vi "SRQ Mode.vi"(8 "error in (no error)":errorcluster, 9 "srq (0:off)":u16(ring) items=["off", "all output faults", "error conditions", "both fault and error conditions"], 11 "VISA resource name":refnum<visa-resource-name>) -> (0 "error out":errorcluster, 3 "VISA resource name out":refnum<visa-resource-name>)   [LabVIEW 2020, in "Agilent 6XXX Series.lvlib"]
doc: "This function enables or disables the SRQ feature for the HP662XA series only."
uses:
  <instrlib>/Agilent 6XXX Series/Agilent 6XXX Series.lvlib
panel:
  # "HP662XA series only"
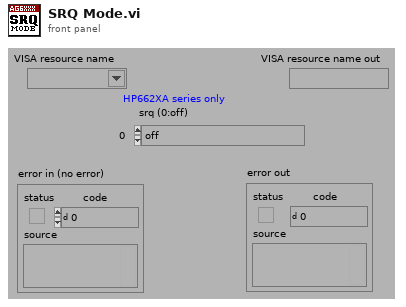
[diagram p1: front panel]
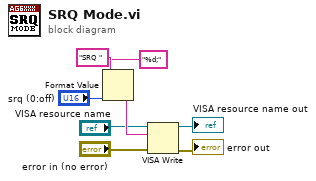
[diagram p0: block diagram]
diagram:
  n1 = Format Value(string ("")="SRQ ", format string="%d;", value (0)="srq (0:off)") -> (output string=w5:string)
  n2 = VISA Write(VISA resource name="VISA resource name", write buffer=w5, error in (no error)="error in (no error)") -> (VISA resource name out=→"VISA resource name out":refnum<visa-resource-name>, error out=→"error out":errorcluster)  [unwired: 1 out]
